vi "digitsToInt.vi"(8 "Numeric":u8, 11 "Numeric 2":u8) -> (3 "x+y":u8)   [LabVIEW 2019]
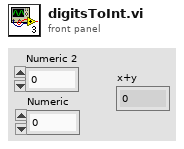
[diagram p1: front panel]
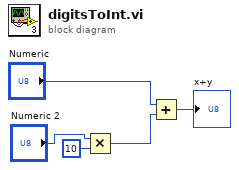
[diagram p0: block diagram]
diagram:
  n1 = Multiply(x="Numeric 2", y=u8 10) -> (x*y=w2:u8)
  n2 = Add(x="Numeric", y=w2) -> (x+y=→"x+y":u8)
